vi "Untitled 2.vi"() -> ()   [LabVIEW 2012]
panel:
  in  "Boolean":bool
  out "Numeric 2":i32
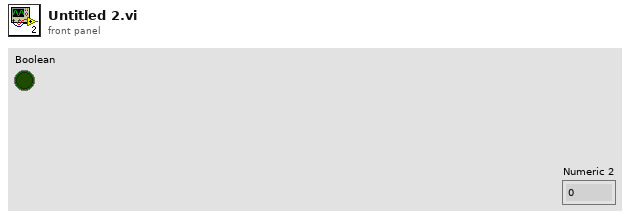
[diagram p1: front panel]
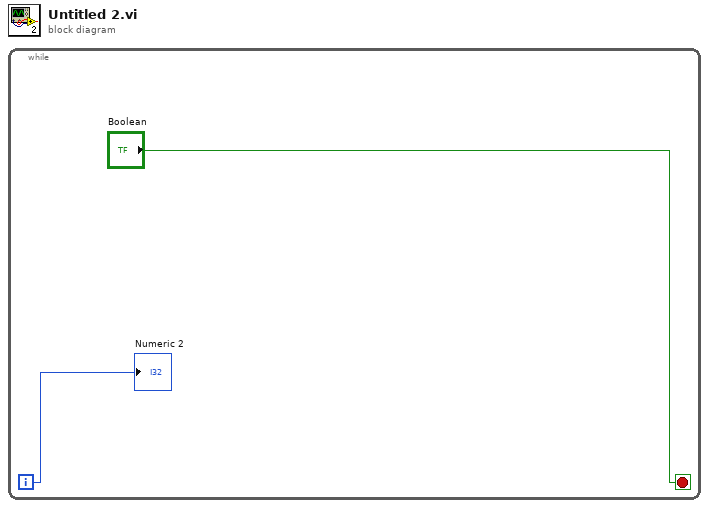
[diagram p0: block diagram]
diagram:
  n1 = while {
    i -> [w2]
    stop <- "Boolean" stop-if-true
    "Numeric 2" <- w2
  }
